vi "CalculateDelay_From_Fi_korr_5761.vi"(8 "input valid":bool=TRUE, 9 "fi_korr ch3":fxp<+/-,32,4>, 10 "fi_korr ch1":fxp<+/-,32,4>, 11 "Data in":fxp<+/-,32,14>[](array[numeric])=[0.0, 0.0, 0.0, 0.0, 0.0, 0.0, 0.0, 0.0]) -> (0 "output valid":bool, 3 "Data out":fxp<+/-,32,14>[](array[numeric]))   [LabVIEW 2018]
doc: "Calculates various combinations on I_in, Q_in and cos(fi) and sin(fi) to be used later to delay the output signal"
uses:
  <vilib>/rvi/FXPMathLib/FxpSinAndCos/subVIs/nifxpmath_SinAndCos_SimConfig.ctl
  <vilib>/rvi/FXPMathLib/FxpSinAndCos/simVIs/DllFxpSinAndCosTemp_sub.vi
  <vilib>/rvi/FXPMathLib/FxpSinAndCos/XNode/nifxpmath_SinAndCos.xnode
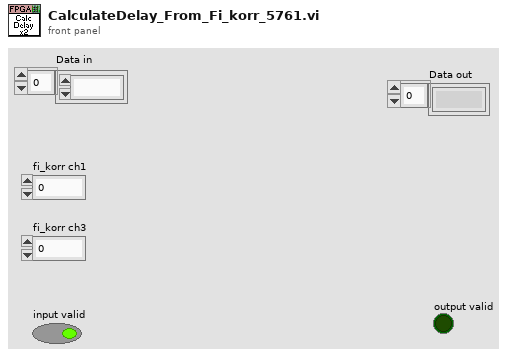
[diagram p1: front panel]
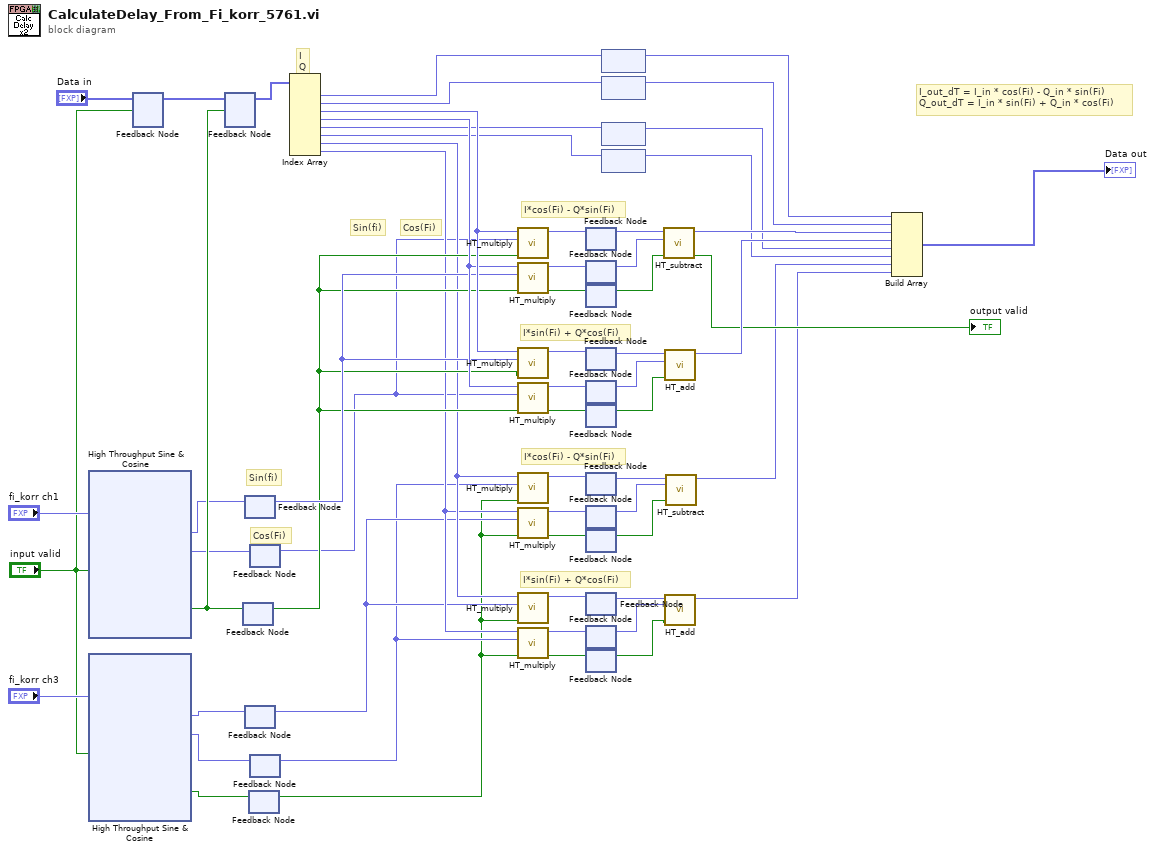
[diagram p0: block diagram]
diagram:
  # "I*sin(Fi) + Q*cos(Fi)"
  # "I*cos(Fi) - Q*sin(Fi)"
  # "Cos(Fi)"
  # "Sin(fi)"
  # "Cos(Fi)"
  # "Sin(fi)"
  # "I_out_dT = I_in * cos(Fi) - Q_in * sin(Fi)\nQ_out_dT = I_in * sin(Fi) + Q_in * cos(Fi)"
  # "I*sin(Fi) + Q*cos(Fi)"
  # "I\nQ"
  # "I*cos(Fi) - Q*sin(Fi)"
  n1 = xnode "High Throughput Sine & Cosine"("x (pi)"="fi_korr ch1", "input valid"="input valid") -> ("sin(x)"=w26:fxp<+/-,16,2>, "cos(x)"=w25:fxp<+/-,16,2>, "output valid"=w27:bool)  [unwired: 1 in, 1 out]
  n2 = xnode "High Throughput Sine & Cosine"("x (pi)"="fi_korr ch3", "input valid"="input valid") -> ("sin(x)"=w7:fxp<+/-,16,2>, "cos(x)"=w6:fxp<+/-,16,2>, "output valid"=w5:bool)  [unwired: 1 in, 1 out]
  n3 = feedback #1() -> (w22:fxp<+/-,32,14>[])  [unwired: 1 in]
  n4 = feedback-in #1("Data in", "input valid") -> ()
  n5 = feedback #2() -> (w24:fxp<+/-,32,14>[])  [unwired: 1 in]
  n6 = feedback-in #2(w22, w27) -> ()
  n7 = feedback #3() -> (w28:bool)  [unwired: 1 in]
  n8 = feedback-in #3(w27) -> ()
  n9 = feedback #4() -> (w30:fxp<+/-,16,2>)  [unwired: 1 in]
  n10 = feedback-in #4(w26) -> ()
  n11 = feedback #5() -> (w4:fxp<+/-,16,2>)  [unwired: 1 in]
  n12 = feedback-in #5(w7) -> ()
  n13 = feedback #6() -> (w1:bool)  [unwired: 1 in]
  n14 = feedback-in #6(w5) -> ()
  n15 = feedback #7() -> (w2:fxp<+/-,16,2>)  [unwired: 1 in]
  n16 = feedback-in #7(w25) -> ()
  n17 = feedback #8() -> (w3:fxp<+/-,16,2>)  [unwired: 1 in]
  n18 = feedback-in #8(w6) -> ()
  n19 = Index Array(array=w24) -> (element #1=w19:fxp<+/-,32,14>, element #2=w18:fxp<+/-,32,14>, element #3=w54:fxp<+/-,32,14>, element #4=w53:fxp<+/-,32,14>, element #5=w17:fxp<+/-,32,14>, element #6=w16:fxp<+/-,32,14>, element #7=w21:fxp<+/-,32,14>, element #8=w20:fxp<+/-,32,14>)  [unwired: 8 in]
  n20 = call "HT_multiply.vi"("input valid"=w28, "y"=w2, "x"=w54) -> ("x*y"=w60:fxp<+/-,32,14>)  [unwired: 7 in, 1 out]
  n21 = call "HT_multiply.vi"("input valid"=w28, "y"=w30, "x"=w53) -> ("output valid"=w58:bool, "x*y"=w59:fxp<+/-,32,14>)  [unwired: 7 in]
  n22 = call "HT_multiply.vi"("input valid"=w28, "y"=w30, "x"=w54) -> ("x*y"=w55:fxp<+/-,32,14>)  [unwired: 7 in, 1 out]
  n23 = call "HT_multiply.vi"("input valid"=w28, "y"=w2, "x"=w53) -> ("output valid"=w57:bool, "x*y"=w56:fxp<+/-,32,14>)  [unwired: 7 in]
  n24 = call "HT_multiply.vi"("input valid"=w1, "y"=w3, "x"=w21) -> ("x*y"=w46:fxp<+/-,32,14>)  [unwired: 7 in, 1 out]
  n25 = call "HT_multiply.vi"("input valid"=w1, "y"=w4, "x"=w20) -> ("output valid"=w48:bool, "x*y"=w47:fxp<+/-,32,14>)  [unwired: 7 in]
  n26 = call "HT_multiply.vi"("input valid"=w1, "y"=w4, "x"=w21) -> ("x*y"=w51:fxp<+/-,32,14>)  [unwired: 7 in, 1 out]
  n27 = call "HT_multiply.vi"("input valid"=w1, "y"=w3, "x"=w20) -> ("output valid"=w49:bool, "x*y"=w50:fxp<+/-,32,14>)  [unwired: 7 in]
  n28 = feedback #9() -> (w35:fxp<+/-,32,14>)  [unwired: 1 in]
  n29 = feedback-in #9(w60) -> ()
  n30 = feedback #10() -> (w31:fxp<+/-,32,14>)  [unwired: 1 in]
  n31 = feedback-in #10(w59) -> ()
  n32 = feedback #11() -> (w32:bool)  [unwired: 1 in]
  n33 = feedback-in #11(w58) -> ()
  n34 = feedback #12() -> (w37:fxp<+/-,32,14>)  [unwired: 1 in]
  n35 = feedback-in #12(w55) -> ()
  n36 = feedback #13() -> (w38:fxp<+/-,32,14>)  [unwired: 1 in]
  n37 = feedback-in #13(w56) -> ()
  n38 = feedback #14() -> (w39:bool)  [unwired: 1 in]
  n39 = feedback-in #14(w57) -> ()
  n40 = feedback #15() -> (w42:fxp<+/-,32,14>)  [unwired: 1 in]
  n41 = feedback-in #15(w46) -> ()
  n42 = feedback #16() -> (w41:fxp<+/-,32,14>)  [unwired: 1 in]
  n43 = feedback-in #16(w47) -> ()
  n44 = feedback #17() -> (w40:bool)  [unwired: 1 in]
  n45 = feedback-in #17(w48) -> ()
  n46 = feedback #18() -> (w45:fxp<+/-,32,14>)  [unwired: 1 in]
  n47 = feedback-in #18(w51) -> ()
  n48 = feedback #19() -> (w44:fxp<+/-,32,14>)  [unwired: 1 in]
  n49 = feedback-in #19(w50) -> ()
  n50 = feedback #20() -> (w43:bool)  [unwired: 1 in]
  n51 = feedback-in #20(w49) -> ()
  n52 = feedback #21() -> (w15:fxp<+/-,32,14>)  [unwired: 1 in]
  n53 = feedback-in #21(w19) -> ()
  n54 = feedback #22() -> (w14:fxp<+/-,32,14>)  [unwired: 1 in]
  n55 = feedback-in #22(w18) -> ()
  n56 = feedback #23() -> (w11:fxp<+/-,32,14>)  [unwired: 1 in]
  n57 = feedback-in #23(w17) -> ()
  n58 = feedback #24() -> (w10:fxp<+/-,32,14>)  [unwired: 1 in]
  n59 = feedback-in #24(w16) -> ()
  n60 = call "HT_subtract.vi"("input valid"=w32, "y"=w31, "x"=w35) -> ("output valid"=→"output valid":bool, "x+y"=w34:fxp<+/-,32,14>)  [unwired: 7 in]
  n61 = call "HT_add.vi"("input valid"=w39, "y"=w38, "x"=w37) -> ("x+y"=w36:fxp<+/-,32,14>)  [unwired: 7 in, 1 out]
  n62 = call "HT_add.vi"("input valid"=w43, "y"=w44, "x"=w45) -> ("x+y"=w13:fxp<+/-,32,14>)  [unwired: 7 in, 1 out]
  n63 = call "HT_subtract.vi"("input valid"=w40, "y"=w41, "x"=w42) -> ("x+y"=w12:fxp<+/-,32,14>)  [unwired: 7 in, 1 out]
  n64 = Build Array(w15, w14, w34, w36, w11, w10, w12, w13) -> (→"Data out":fxp<+/-,32,14>[])
